vi "Save Menu.vi"(8 "error in (no error)":errorcluster, 9 "Menu ref":refnum<vi>, 10 "File path":path, 11 "Monitor-Pulse in":refnum<class "Application Controller.lvclass">) -> (0 "error out":errorcluster, 1 "Section out":string, 2 "File path out":path, 3 "Monitor-Pulse out":refnum<class "Application Controller.lvclass">)   [LabVIEW 2016, in "Application Controller.lvclass"]
uses:
  Application Controller.lvclass
  C:/github/LabActor/Template Module/Template Module.lvclass
  NHMFL_Core/Libraries/Queued Listbox/Queued Listbox.xctl
  Template Module/Template Module.lvclass/Template Module.ctl
  Template Module/Read Name.vi
  <vilib>/Utility/config.llb/NI_LVConfig.lvlib
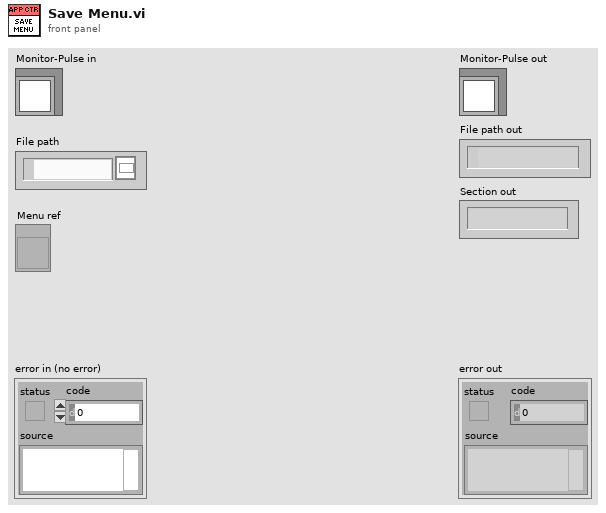
[diagram p1: front panel]
types:
  T1 = typedef "NI_LVConfig.lvlib/Config Data RefNum.ctl" = refnum<k1>
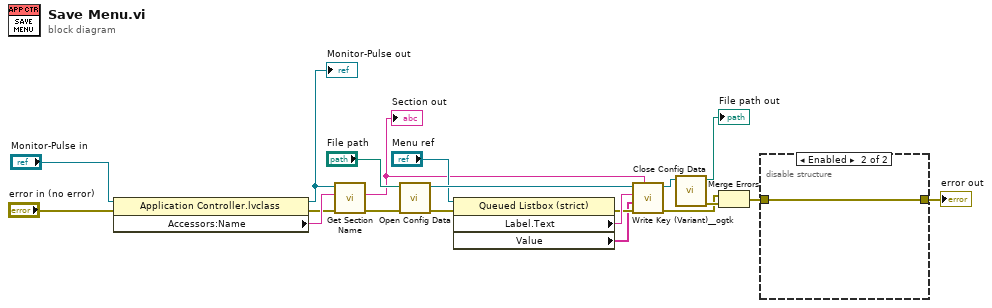
[diagram p0: block diagram]
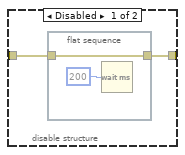
[diagram p2: hidden frame]
diagram:
  n1 = property class="Application Controller.lvclass"(reference="Monitor-Pulse in", error in="error in (no error)") -> (reference out=w1:refnum<class "Application Controller.lvclass">, error out=w6:errorcluster, "Accessors:Name"=w14:string)
  "Monitor-Pulse out" <- w1
  n2 = call "Get Section Name.vi"("Error In"=w6, "Object name"=w14, "object"=w1) -> ("Error Out"=w10:errorcluster, "Section out"=w2:string)  [unwired: 7 in]
  "Section out" <- w2
  n3 = call <vilib>:"Open Config Data.vi"("error in (no error)"=w10, "configuration file path"="File path") -> ("error out"=w9:errorcluster, "refnum"=w20:T1)  [unwired: 7 in, 1 out]
  n4 = property class="Queued Listbox (strict)"(reference="Menu ref", error in=w9) -> (error out=w5:errorcluster, "Label.Text"=w16:string, "Value"=w4:string[])  [unwired: 1 out]
  n5 = call <userlib>:"Write Key (Variant)__ogtk.vi"("section"=w2, "error in (no error)"=w5, "key-value"=w4, "key (optional)"=w16, "refnum"=w20) -> ("error out"=w18:errorcluster, "refnum out"=w17:T1)  [unwired: 5 in]
  n6 = call <vilib>:"Close Config Data.vi"("refnum"=w17) -> ("error out"=w19:errorcluster, "file path"=→"File path out":path)  [unwired: 9 in]
  n7 = Merge Errors(w18, w19) -> (w11:errorcluster)
  n8 = disable-structure shown="Enabled" {
    disable-tunnel: w11 -> [w22 w25]
    disable-tunnel: [w21 w25] -> w8
    frame Disabled {
      n9 = flat-sequence {
        tunnel: w22 -> [w24]
        tunnel: [w24] -> w21
        frame #0 {
          n10 = Wait (ms)(milliseconds to wait=u32 200) -> ()  [unwired: 1 out]
        }
      }
    }
    frame Enabled {
    }
  }
  "error out" <- w8
